vi "appendRawDataToWaveform.vi"(8 "ErrorIn":errorcluster, 9 "Tacho signal In":waveform(dbl), 10 "RawAccelerationData":dbl[][](array[numeric]), 11 "AccelerationDataIn":waveform(dbl)[](array[waveform])=[{"t0"=timestamp(0 s since 1904-01-01), "dt"=0.0, "Y"=[]}, {"t0"=timestamp(0 s since 1904-01-01), "dt"=0.0, "Y"=[]}, {"t0"=timestamp(0 s since 1904-01-01), "dt"=0.0, "Y"=[]}]) -> (0 "ErrorOut":errorcluster, 2 "Tacho signal Out":waveform(dbl), 3 "AccelerationDataOut":waveform(dbl)[](array[waveform]))   [LabVIEW 2019]
uses:
  <vilib>/Waveform/WDTOps.llb/WDT Append Waveforms DBL.vi
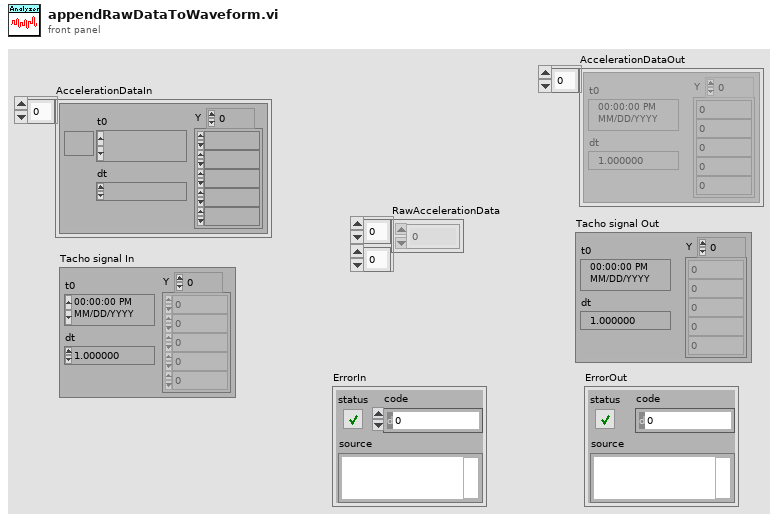
[diagram p1: front panel]
types:
  T1 = typedef "AnalyzerSettings.ctl" = cluster{"Create NS Timeout Code":i32, "Destroy NS Timeout Code":i32, "All threads":T2[], "Connected to app?":bool, "AnalysisSettings":T3}
  T2 = typedef "AThreads.ctl" = enum16{"UI", "analyzeAccelerationData", "aquireAccelerationData", "communicateWebServices", "TDMSmanager", "aquireTachoSignal"}
  T3 = typedef "AnalysisSettings.ctl" = cluster{"Fault Thresholds":T4, "Analysis series name":string, "Save data analysis?":bool, "F-Band Size":i32, "OrderAnalysis?":bool, "Accelerometer":T6, "fs [Hz]":dbl, "Pulse per revolution":u16, "FFT-Parameters":cluster{"averaging mode":enum16{"No averaging", "Vector averaging", "RMS averaging", "Peak hold"}, "weighting mode":enum16{"Linear", "Exponential"}, "number of averages":u32}, "O-WindowPowerSpectrum":u32, "O-SpectrumAveraging":enum16{"No averaging", "Vector averaging", "RMS averaging", "Peak hold"}, "O-MaxOrder":dbl, "O-Resolution":dbl, "O-BandSize":dbl, "FrameLength [s]":dbl, "Aq.FrameLength [ms]":i64, "FilterOrder":i32, "Sensitivity [V/g]":dbl[]}
  T4 = typedef "Thresholds.ctl" = cluster{"Parameters labels":T5[], "Parameters thresholds":dbl[], "Freqs and thresholds":dbl[][], "Orders and thresholds":dbl[][]}
  T5 = typedef "FaultParameter.ctl" = enum16{"Kurtosis", "RMS", "Crest factor"}
  T6 = typedef "Accelerometer.ctl" = enum16{"None", "MPU6050", "MMA7351"}
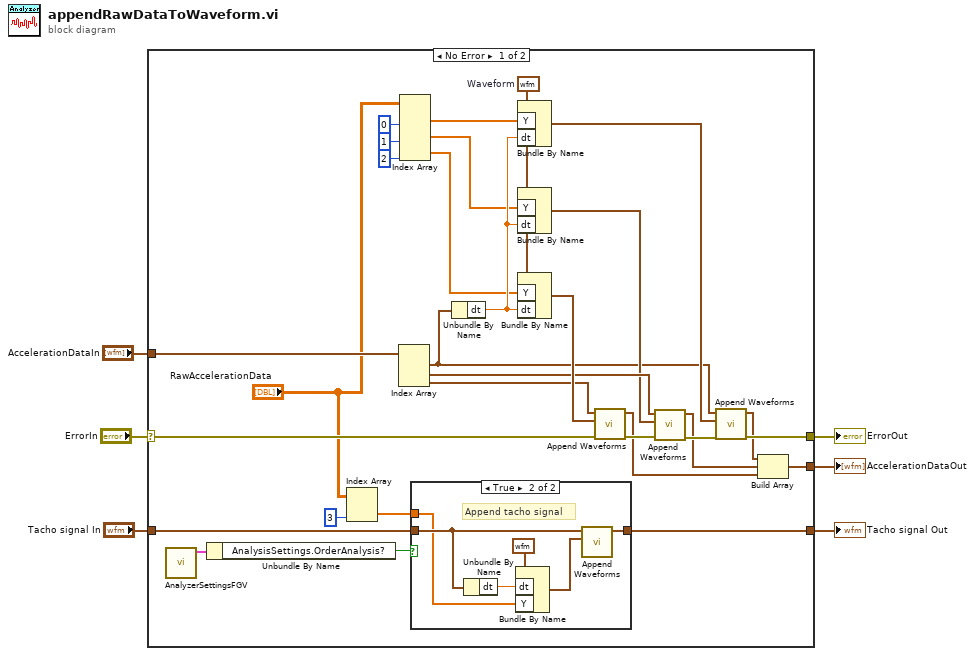
[diagram p0: block diagram]
diagram:
  n1 = case shown="No Error" "ErrorIn" {
    selector: "ErrorIn" -> [w16 w46]
    tunnel: [w30 w46] -> w5
    tunnel: "AccelerationDataIn" -> [w24 w44]
    tunnel: [w23 w44] -> w3
    tunnel: "Tacho signal In" -> [w20 w45]
    tunnel: [w19 w45] -> w1
    frame No Error {
      w36 = waveform(dbl) {"t0"=timestamp(0 s since 1904-01-01), "dt"=0.0, "Y"=[]}  # Waveform
      n2 = call "AnalyzerSettingsFGV.vi"() -> ("AnalyzerSettingsOut"=w18:T1)  [unwired: 11 in]
      n3 = Unbundle By Name(w18) -> ("AnalysisSettings.OrderAnalysis?"=w17:bool)
      n4 = Index Array(array="RawAccelerationData", index (col)=3 ("index (row)")) -> (element=w12:dbl[])  [unwired: 1 in]
      n5 = Index Array(array=w24) -> (element #1=w22:waveform(dbl), element #2=w33:waveform(dbl), element #3=w34:waveform(dbl))  [unwired: 3 in]
      n6 = Index Array(array="RawAccelerationData", index (col) #1=0 ("disabled index (col)"), index (col) #2=1 ("index (col)"), index (col) #3=2 ("index (col)")) -> (element #1=w15:dbl[], element #2=w14:dbl[], element #3=w13:dbl[])  [unwired: 3 in]
      n7 = case shown="True" w17 {
        tunnel: w20 -> [w37 w40]
        tunnel: [w37 w39] -> w19
        tunnel: w12 -> [_ w38]
        frame False {
        }
        frame True {
          # "Append tacho signal"
          n8 = Unbundle By Name(w40) -> ("dt"=w42:dbl)
          n9 = Bundle By Name(cluster=waveform(dbl) {"t0"=timestamp(0 s since 1904-01-01), "dt"=0.0, "Y"=[]} ("analog tacho signal"), "dt"=w42, "Y"=w38) -> (w41:waveform(dbl))
          n10 = call-poly <vilib>:"Append Waveforms.vi"("waveform B"=w41, "waveform A"=w40) -> ("waveform out"=w39:waveform(dbl))  [unwired: 8 in, 1 out]
        }
      }
      n11 = Unbundle By Name(w22) -> ("dt"=w21:dbl)
      n12 = Bundle By Name(cluster=w36, "Y"=w15, "dt"=w21) -> (w28:waveform(dbl))
      n13 = Bundle By Name(cluster=w36, "Y"=w14, "dt"=w21) -> (w29:waveform(dbl))
      n14 = Bundle By Name(cluster=w36, "Y"=w13, "dt"=w21) -> (w35:waveform(dbl))
      n15 = call-poly <vilib>:"Append Waveforms.vi"("error in (no error)"=w16, "waveform B"=w35, "waveform A"=w34) -> ("error out"=w32:errorcluster, "waveform out"=w27:waveform(dbl))  [unwired: 7 in]
      n16 = call-poly <vilib>:"Append Waveforms.vi"("error in (no error)"=w32, "waveform B"=w29, "waveform A"=w33) -> ("error out"=w31:errorcluster, "waveform out"=w26:waveform(dbl))  [unwired: 7 in]
      n17 = call-poly <vilib>:"Append Waveforms.vi"("error in (no error)"=w31, "waveform B"=w28, "waveform A"=w22) -> ("error out"=w30:errorcluster, "waveform out"=w25:waveform(dbl))  [unwired: 7 in]
      n18 = Build Array(w25, w26, w27) -> (w23:waveform(dbl)[])
    }
    frame Error {
    }
  }
  "ErrorOut" <- w5
  "AccelerationDataOut" <- w3
  "Tacho signal Out" <- w1
